vi "lib Find String Matches in Array.vi"(8 "error in (no error)":errorcluster, 9 "ID":i32[](array[numeric]), 10 "Search Strings":string[](array[string]), 11 "All Strings":string[](array[string])) -> (0 "error out":errorcluster, 1 "ID Out":i32[](array[numeric]), 3 "Matches":string[](array[string]))   [LabVIEW 2014]
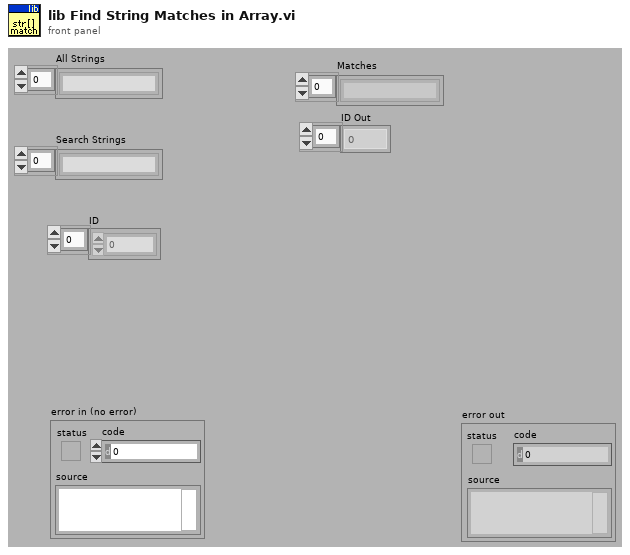
[diagram p1: front panel]
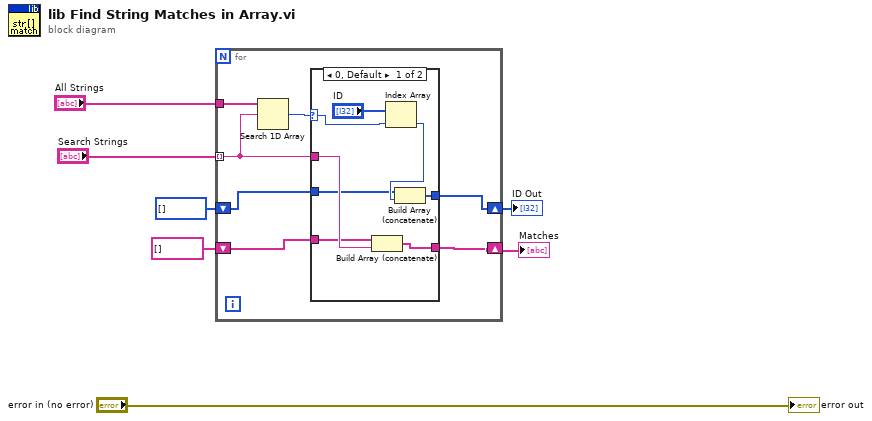
[diagram p0: block diagram]
diagram:
  n1 = for {
    tunnel: "Search Strings" -> [w12] mode=indexing
    tunnel: "All Strings" -> [w14]
    shift-right: [w11] -> w3
    shift-left: string[] [] -> [w10]
    shift-right: [w9] -> w1
    shift-left: i32[] [] -> [w8]
    n2 = Search 1D Array(1D array=w14, element=w12) -> (index of element=w13:i32)  [unwired: 1 in]
    n3 = case shown="0, Default" w13 {
      selector: w13 -> [w18 _]
      tunnel: w12 -> [w22 _]
      tunnel: [w21 w24] -> w11
      tunnel: w10 -> [w20 w24]
      tunnel: [w16 w23] -> w9
      tunnel: w8 -> [w15 w23]
      frame 0, Default {
        n4 = Build Array (concatenate)(w20, w22) -> (w21:string[])
        n5 = Index Array(array="ID", index=w18) -> (element=w17:i32)
        n6 = Build Array (concatenate)(w15, w17) -> (w16:i32[])
      }
      frame -1 {
      }
    }
  }
  "Matches" <- w3
  "ID Out" <- w1
  "error out" <- "error in (no error)"
